vi "Rasnik_Gabri.vi"() -> ()   [LabVIEW 2015]
uses:
  GlobalPath.vi
  GlobalData.vi
  <vilib>/Utility/file.llb/Read Delimited Spreadsheet (string).vi
  <vilib>/Utility/file.llb/Write Delimited Spreadsheet (DBL).vi
panel:
  out "all rows 4":string[][](array[string])
  out "all rows 3":string[][](array[string])
  out "appended path 2":path
  in  "Done?":bool
  in  "Stage":string
  in  "driver off":bool caption="Disconnect the driver from the power supply"
  out "text":string
  out "PanelName":string
  out "appended path":path
  out "Y Diff10":dbl
  out "Y Diff9":dbl
  out "Y Diff8":dbl
  out "Y Diff7":dbl
  out "Y Diff6":dbl
  out "Y Diff5":dbl
  out "Y Diff4":dbl
  out "Y Diff3":dbl
  out "Y Diff2":dbl
  out "Y Diff1":dbl
  out "X Diff10":dbl
  out "X Diff9":dbl
  out "X Diff8":dbl
  out "X Diff7":dbl
  out "X Diff6":dbl
  out "X Diff5":dbl
  out "X Diff4":dbl
  out "X Diff3":dbl
  out "X Diff2":dbl
  out "X Diff1":dbl
  out "all rows":string[][](array[string])
  out "Y D10":dbl format="%.2f"
  out "Y D9":dbl format="%.2f"
  out "Y D8":dbl format="%.2f"
  out "Y D7":dbl format="%.2f"
  out "Y D6":dbl format="%.2f"
  out "Y D5":dbl format="%.2f"
  out "Y D4":dbl format="%.2f"
  out "Y D3":dbl format="%.2f"
  out "Y D2":dbl format="%.2f"
  out "Y D1":dbl
  out "X D10":dbl format="%.2f"
  out "X D9":dbl format="%.2f"
  out "X D8":dbl format="%.2f"
  out "X D7":dbl format="%.2f"
  out "X D6":dbl format="%.2f"
  out "X D5":dbl format="%.2f"
  out "X D4":dbl format="%.2f"
  out "X D3":dbl format="%.2f"
  out "X D2":dbl format="%.2f"
  out "X D1":dbl
  out "y 6":string
  out "y 10":string
  out "y 9":string
  out "y 8":string
  out "y 7":string
  out "y 5":string
  out "y 4":string
  out "y 3":string
  out "y 2":string
  out "y 1":string
  out "x 6":string
  out "x 10":string
  out "x 9":string
  out "x 8":string
  out "x 7":string
  out "x 5":string
  out "x 4":string
  out "x 3":string
  out "x 2":string
  out "x 1":string
  out "Script":path
  out "Filename selected":path
  out "standard output":string
  in  "Done?":bool
  in  "Open Program":bool
  in  "c-ccd 3":bool caption="Setup the electronics for the C-CCD reading:\n- make sure the ethernet cables are connected on the minimal heads\n- check that the cables connecting the driver with the muxs are plugged in\n- CONNECT the driver to the power supply and check that it is connected to the LAN\nIf the measurements show -1 in all c-ccds:\nUNPLUG the driver, WAIT a couple of seconds and REPLUG it"
  in  "c-ccd":bool caption="Read the data file"
  # "Rasmask reading from PCBs on stiffback/table"
  # "Type \"Table\" or \"Stiffback\" for the C-CCDs you want to use:"
  # "Run the C-CCD reading program \n(the 10 Rasmasks are automatically read and the data saved)"
  # "Data file reading"
  # "The most recent data file created by the C-CCD program will be opened.\nOnce the \"read data file\" is clicked, the raw data and displacement should appear on the PCB schematics on the bottom."
  # "Raw Data (mm):"
  # "Calibrated position (mm):"
  # "Difference (wrt Reference reading) (um):"
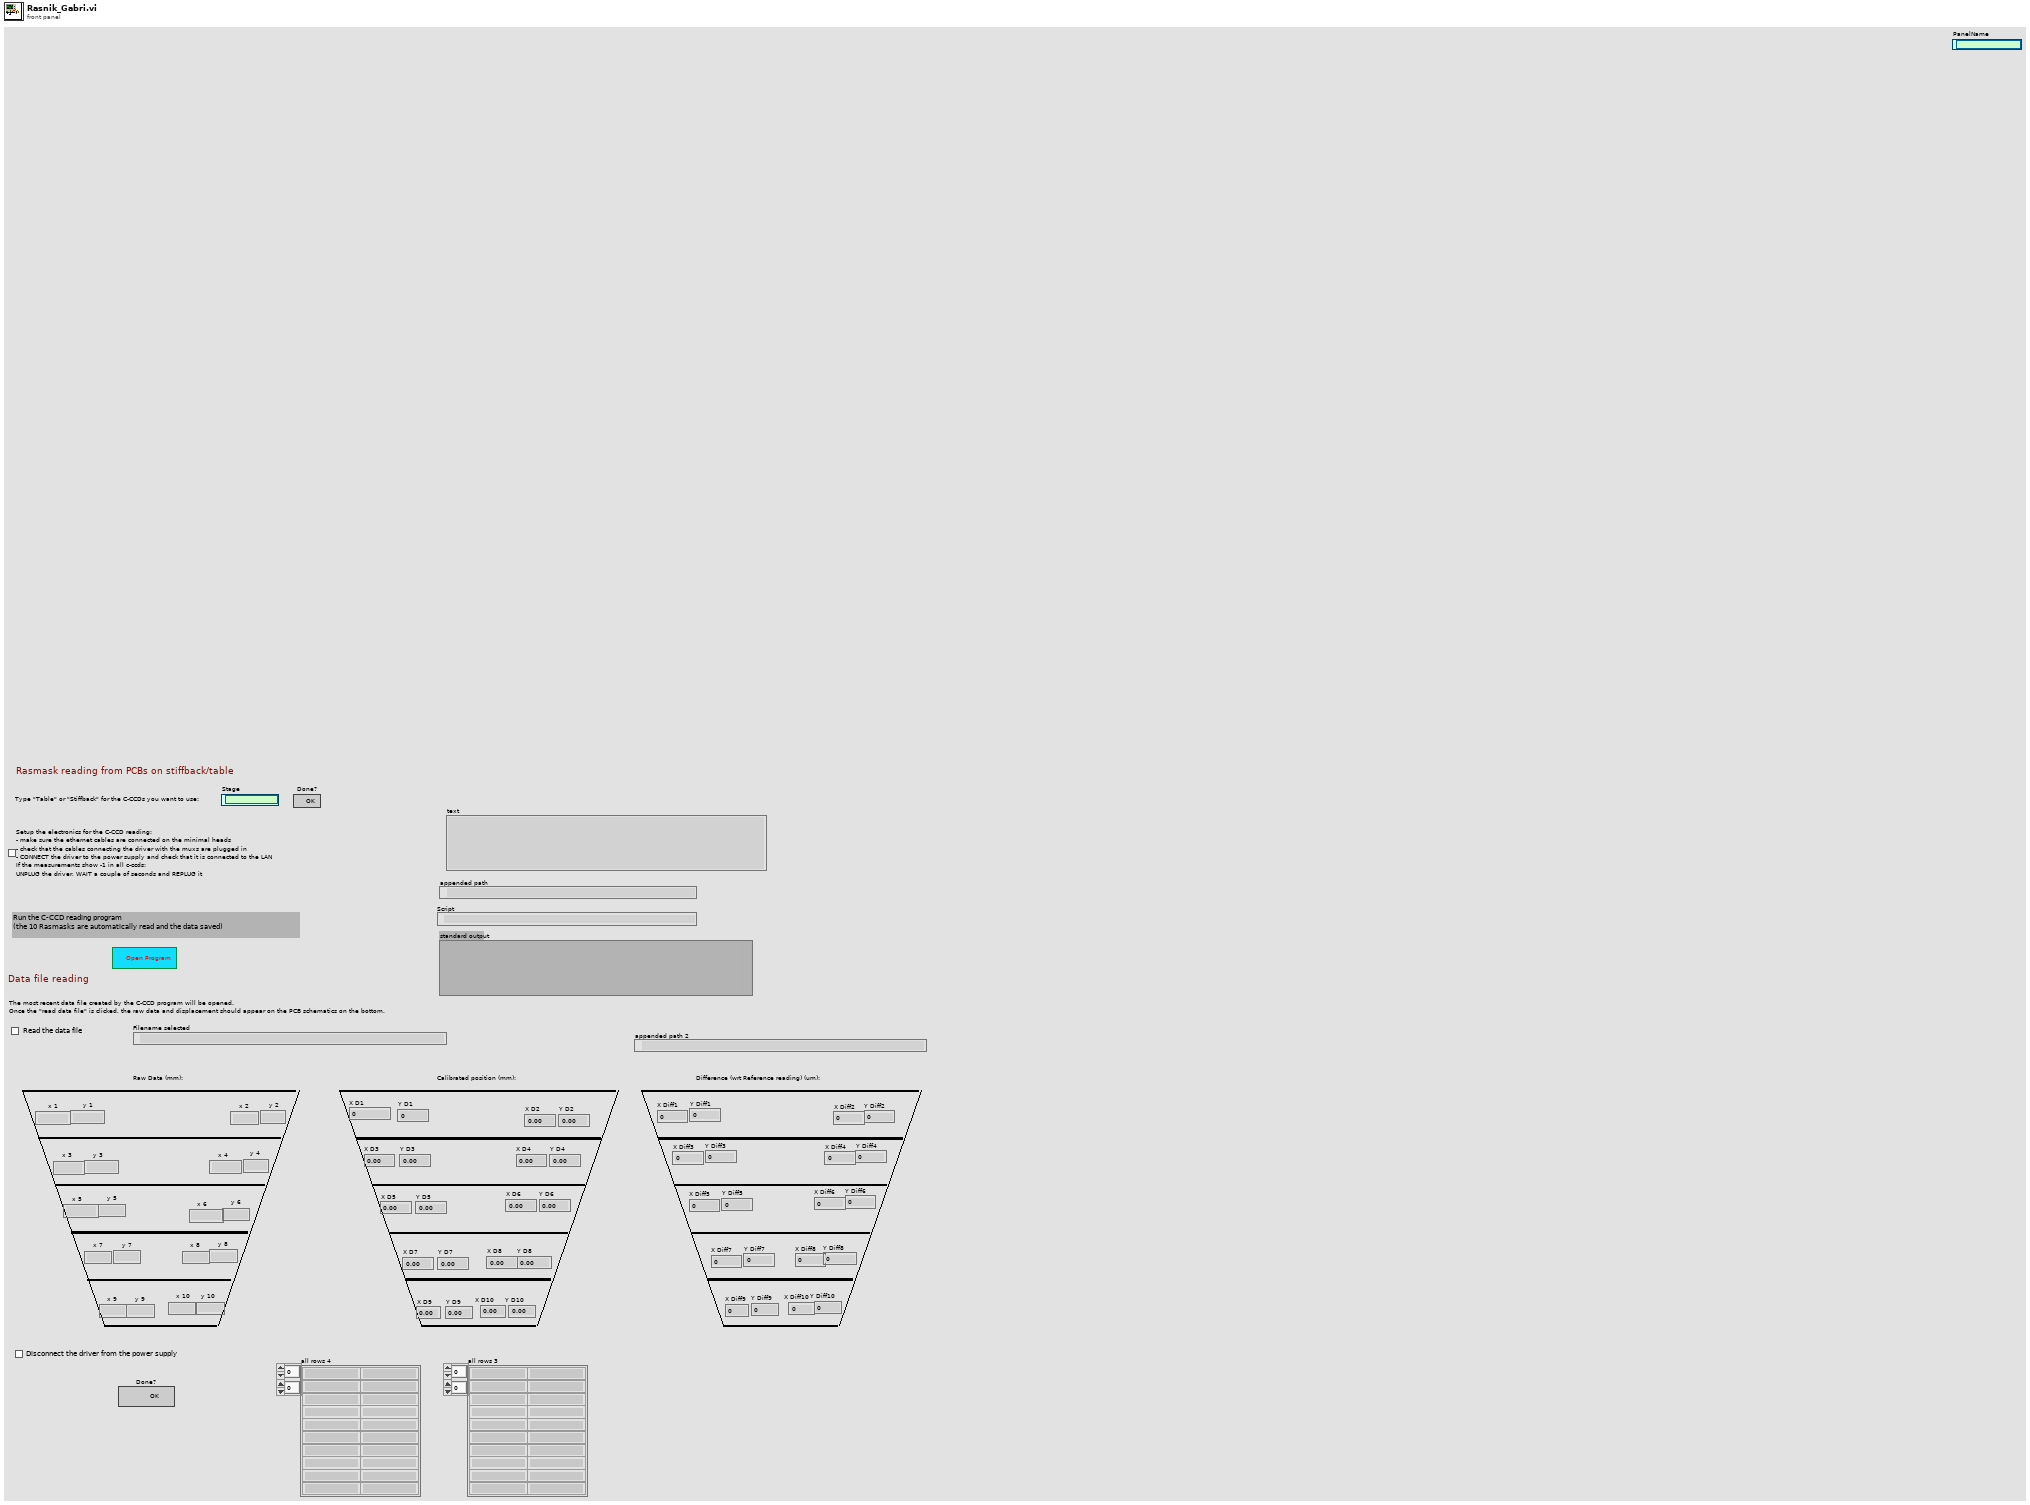
[diagram p1: front panel]
types:
  T1 = enum16{"open", "replace", "create", "open or create", "replace or create", "replace or create with confirmation"}
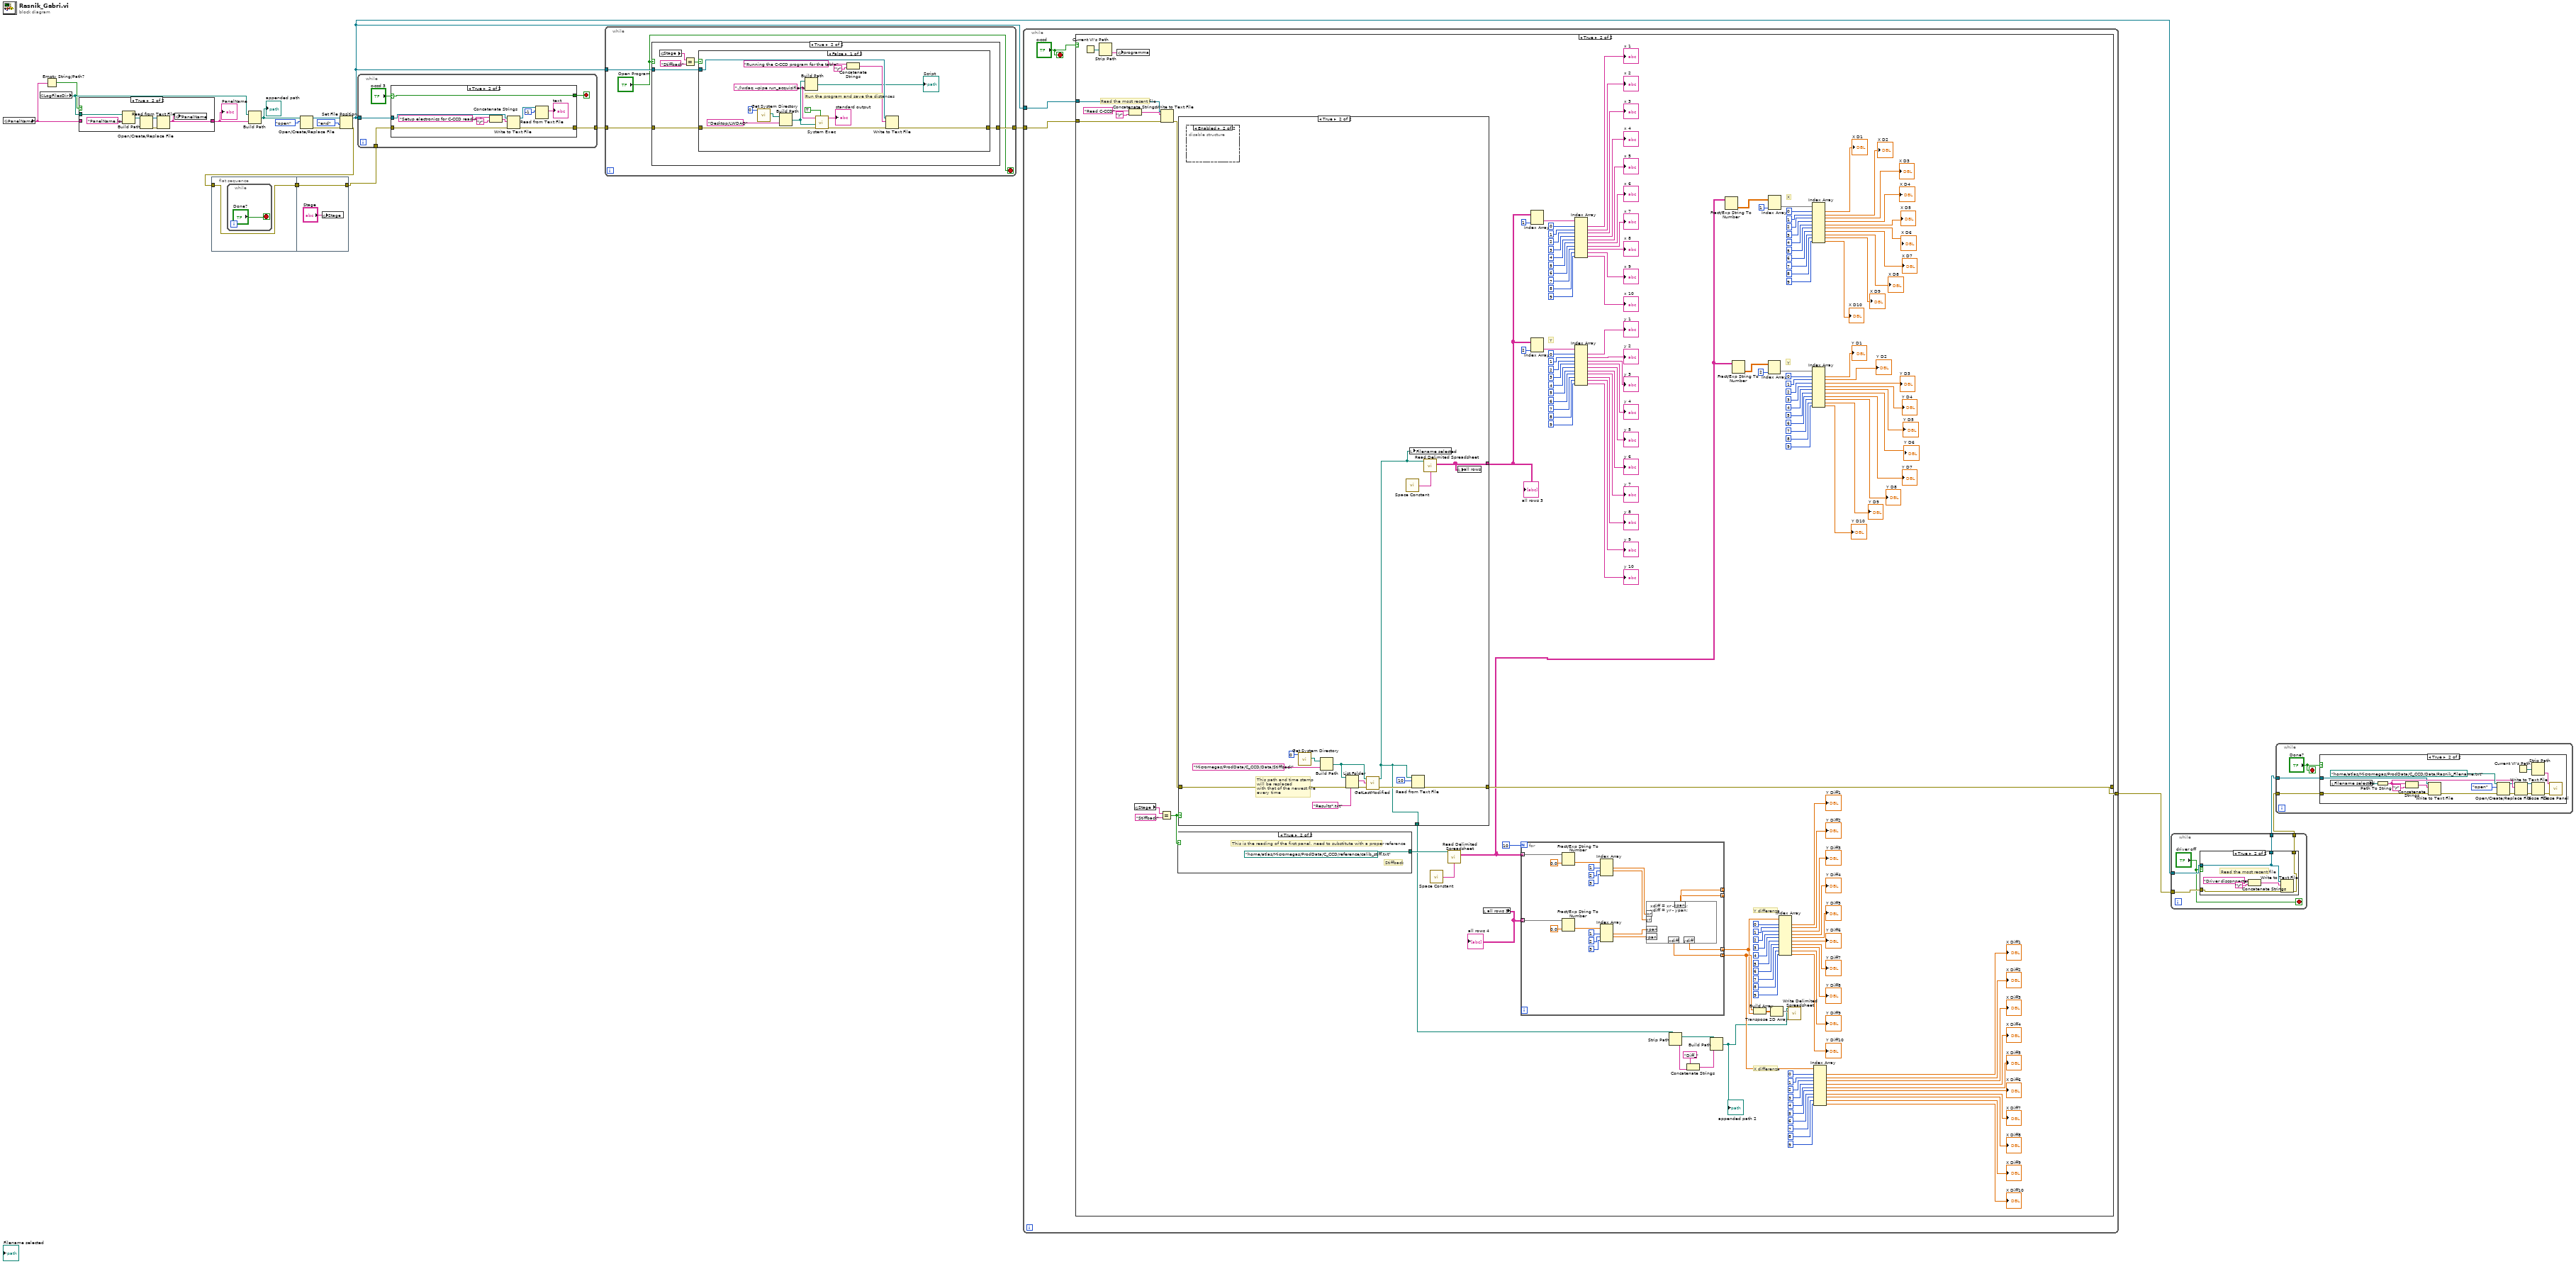
[diagram p0: block diagram]
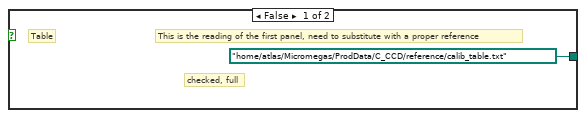
[diagram p5: hidden frame]
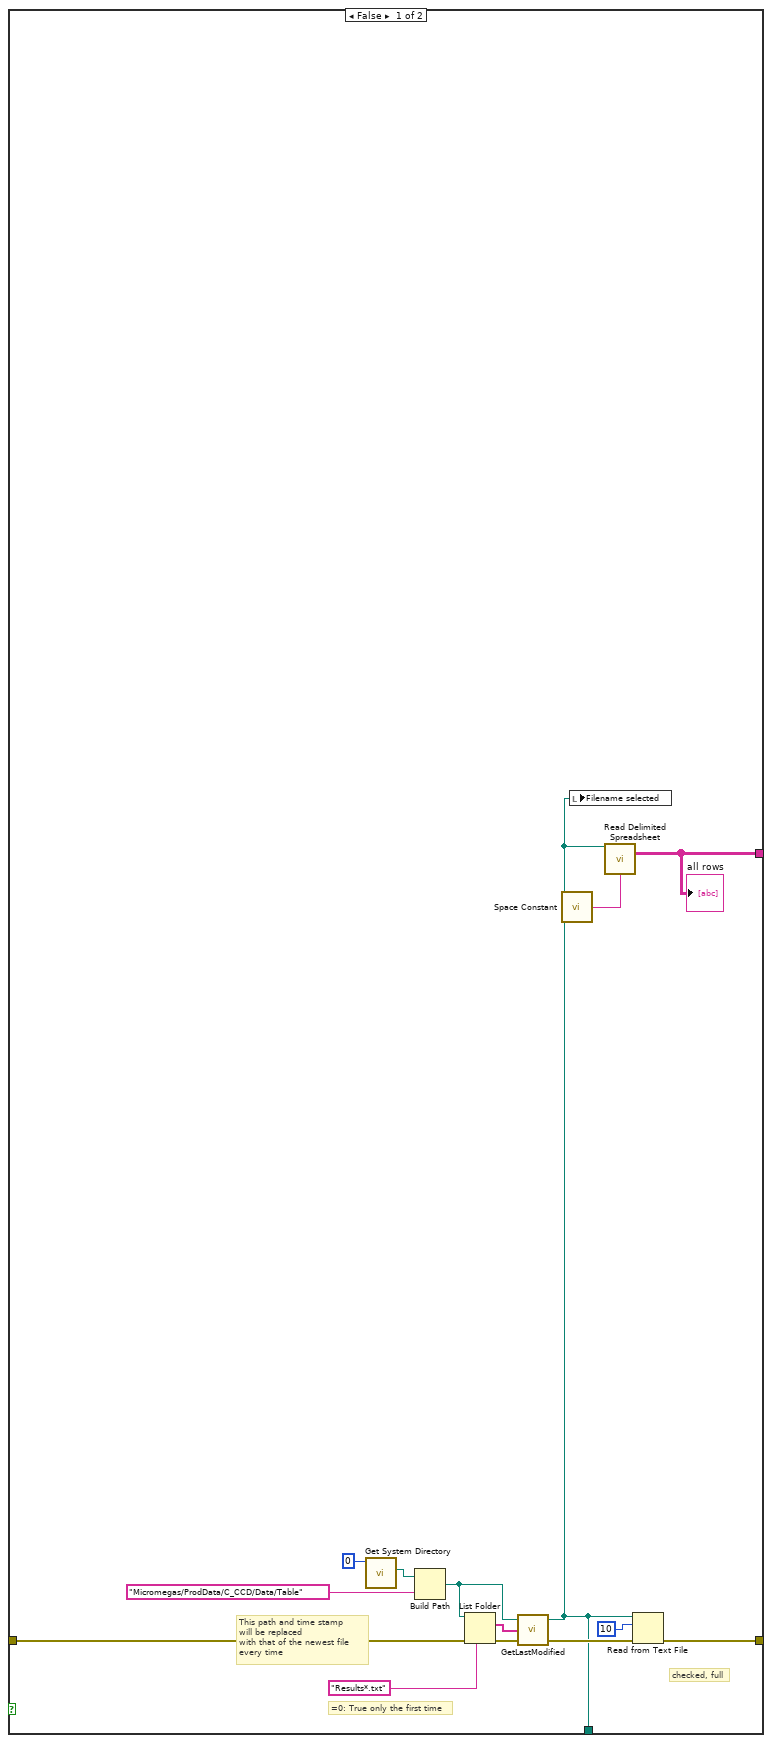
[diagram p6: hidden frame]
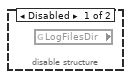
[diagram p7: hidden frame]
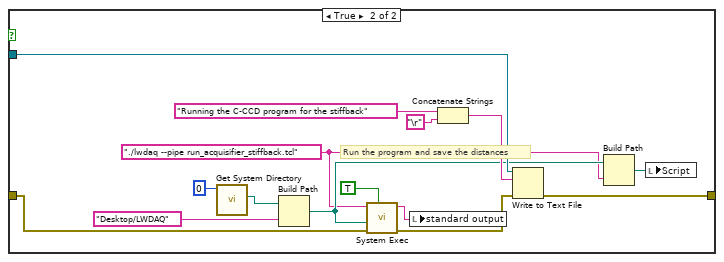
[diagram p10: hidden frame]
diagram:
  n1 = global read "GlobalData.vi" "PanelName"() -> (w14:string)
  n2 = global read "GlobalPath.vi" "LogFilesDir"() -> (w15:path)
  n3 = Empty String/Path?(string/path=w14) -> (empty?=w13:bool)
  n4 = case shown="True" w13 {
    tunnel: w15 -> [_ w25]
    tunnel: [w19 w20] -> w16
    tunnel: w14 -> [w19 _]
    frame False {
    }
    frame True {
      n5 = Build Path(base path=w25, name or relative path="PanelName.log") -> (appended path=w24:path)
      n6 = Open/Create/Replace File(file path (use dialog)=w24) -> (refnum out=w21:refnum<file>, error out=w22:errorcluster)  [unwired: 5 in, 1 out]
      n7 = Read from Text File(file (use dialog)=w21, error in=w22) -> (text=w20:string)  [unwired: 2 in, 3 out]
      n8 = global write "GlobalData.vi" "PanelName"(w20) -> ()
    }
  }
  "PanelName" <- w16
  n9 = flat-sequence {
    tunnel: w3 -> [w26]
    tunnel: [w26] -> w2
    tunnel: [w28] -> w1
    tunnel: w2 -> [w28]
    frame #0 {
      n10 = while {
        stop <- "Done?" stop-if-true
      }
    }
    frame #1 {
      n11 = global write "GlobalData.vi" "Stage"("Stage") -> ()
    }
  }
  n12 = Build Path(base path=w15, name or relative path=w16) -> (appended path=w8:path)
  "appended path" <- w8
  n13 = Open/Create/Replace File(file path (use dialog)=w8, operation (0:open)=T1."open") -> (refnum out=w11:refnum<file>, error out=w12:errorcluster)  [unwired: 4 in, 1 out]
  n14 = Set File Position(refnum=w11, from (0:start)=enum16{"start", "end", "current"}."end", error in=w12) -> (refnum out=w7:refnum<file>, error out=w3:errorcluster)  [unwired: 1 in]
  n15 = while {
    tunnel: w7 -> [w33]
    tunnel: [w31] -> w17
    tunnel: w1 -> [w30]
    stop <- w32 stop-if-true
    n16 = case shown="True" "c-ccd 3" {
      selector: "c-ccd 3" -> [w36 w43]
      tunnel: [w35 w44] -> w31
      tunnel: w33 -> [_ w41]
      tunnel: [w36 w43] -> w32
      tunnel: w30 -> [w35 w42]
      frame False {
      }
      frame True {
        n17 = Concatenate Strings("Setup electronics for C-CCD reading", "\r") -> (w40:string)
        n18 = Write to Text File(file (use dialog)=w41, text=w40, error in=w42) -> (refnum out=w39:refnum<file>, error out=w44:errorcluster)  [unwired: 1 in, 1 out]
        n19 = Read from Text File(file (use dialog)=w39, count=-1) -> (text=→"text":string)  [unwired: 2 in, 3 out]
      }
    }
  }
  n20 = while {
    tunnel: w7 -> [w48]
    tunnel: w17 -> [w50]
    tunnel: [w49] -> w18
    stop <- "Open Program" stop-if-true
    n21 = case shown="True" "Open Program" {
      tunnel: w50 -> [w51 w54]
      tunnel: [w51 w53] -> w49
      tunnel: w48 -> [_ w52]
      frame False {
      }
      frame True {
        n22 = global read "GlobalData.vi" "Stage"() -> (w56:string)
        n23 = Equal?(x=w56, y="Stiffback") -> (x = y?=w55:bool)
        n24 = case shown="False" w55 {
          tunnel: w54 -> [w69 w84]
          tunnel: [w67 w82] -> w53
          tunnel: w52 -> [w66 w81]
          frame False {
            w59 = "./lwdaq --pipe run_acquisifier.tcl"
            # "Run the program and save the distances"
            n25 = call <vilib>:"Get System Directory.vi"("system directory type"=0) -> ("system directory"=w64:path)  [unwired: 10 in]
            n26 = Build Path(base path=w64, name or relative path="Desktop/LWDAQ") -> (appended path=w60:path)
            n27 = Build Path(base path=w60, name or relative path=w59) -> (appended path=→"Script":path)
            n28 = call <vilib>:"System Exec.vi"("wait until completion? (T)"=TRUE, "error in (no error)"=w69, "working directory"=w60, "command line"=w59) -> ("error out"=w68:errorcluster, "standard output"=→"standard output":string)  [unwired: 4 in, 2 out]
            n29 = Concatenate Strings("Running the C-CCD program for the table", "\r") -> (w72:string)
            n30 = Write to Text File(file (use dialog)=w66, text=w72, error in=w68) -> (error out=w67:errorcluster)  [unwired: 1 in, 2 out]
          }
          frame True {
            w75 = "./lwdaq --pipe run_acquisifier_stiffback.tcl"
            # "Run the program and save the distances"
            n31 = call <vilib>:"Get System Directory.vi"("system directory type"=0) -> ("system directory"=w78:path)  [unwired: 10 in]
            n32 = Build Path(base path=w78, name or relative path="Desktop/LWDAQ") -> (appended path=w76:path)
            n33 = call <vilib>:"System Exec.vi"("wait until completion? (T)"=TRUE, "error in (no error)"=w84, "working directory"=w76, "command line"=w75) -> ("error out"=w83:errorcluster, "standard output"=w73:string)  [unwired: 4 in, 2 out]
            n34 = local write "standard output"(w73) -> ()
            n35 = Concatenate Strings("Running the C-CCD program for the stiffback", "\r") -> (w87:string)
            n36 = Write to Text File(file (use dialog)=w81, text=w87, error in=w83) -> (error out=w82:errorcluster)  [unwired: 1 in, 2 out]
            n37 = Build Path(base path=w76, name or relative path=w75) -> (appended path=w74:path)
            n38 = local write "Script"(w74) -> ()
          }
        }
      }
    }
  }
  n39 = while {
    tunnel: w7 -> [w89]
    tunnel: w18 -> [w91]
    tunnel: [w90] -> w6
    stop <- "c-ccd" stop-if-true
    n40 = case shown="True" "c-ccd" {
      tunnel: w91 -> [w92 w243]
      tunnel: [w92 w241] -> w90
      tunnel: w89 -> [_ w240]
      frame False {
      }
      frame True {
        # "X"
        # "Y"
        # "Y differenza"
        # "X differenza"
        # "Y"
        # "Read the most recent file"
        n41 = Current VI's Path() -> (path=w244:path)
        n42 = Strip Path(path=w244) -> (name=w245:string)  [unwired: 1 out]
        n43 = global write "GlobalData.vi" "programma"(w245) -> ()
        n44 = Concatenate Strings("Read C-CCD", "\r") -> (w250:string)
        n45 = global read "GlobalData.vi" "Stage"() -> (w246:string)
        n46 = Equal?(x=w246, y="Stiffback") -> (x = y?=w151:bool)
        n47 = Write to Text File(file (use dialog)=w240, text=w250, error in=w243) -> (error out=w242:errorcluster)  [unwired: 1 in, 2 out]
        n48 = case shown="True" w151 {
          tunnel: [path "/home/atlas/Micromegas/ProdData/C_CCD/reference/calib_table.txt" ("file path (dialog if empty)") path "/home/atlas/Micromegas/ProdData/C_CCD/reference/calib_stiff.txt" ("file path (dialog if empty)")] -> w195
          frame False {
            # "checked, full"
            # "This is the reading of the first panel, need to substitute with a proper reference"
            # "Table"
          }
          frame True {
            # "Stiffback"
            # "This is the reading of the first panel, need to substitute with a proper reference"
          }
        }
        n49 = case shown="True" w151 {
          tunnel: w242 -> [w276 w290]
          tunnel: [w285 w299] -> w241
          tunnel: [w274 w288] -> w216
          tunnel: [w273 w287] -> w94
          frame False {
            # "checked, full"
            # "=0: True only the first time"
            # "This path and time stamp\nwill be replaced\nwith that of the newest file \nevery time"
            n50 = call <vilib>:"Get System Directory.vi"("system directory type"=0) -> ("system directory"=w283:path)  [unwired: 10 in]
            n51 = Build Path(base path=w283, name or relative path="Micromegas/ProdData/C_CCD/Data/Table") -> (appended path=w278:path)
            n52 = List Folder(path=w278, pattern="Results*.txt", error in=w276) -> (filenames=w281:string[], error out=w279:errorcluster)  [unwired: 1 in, 2 out]
            n53 = call "GetLastModified.vi"("error in"=w279, "filenames"=w281, "SearchDir"=w278) -> ("error out"=w280:errorcluster, "Path"=w273:path)  [unwired: 1 out]
            n54 = call <vilib>:"Space Constant.vi"() -> ("String"=w275:string)
            n55 = local write "Filename selected"(w273) -> ()
            n56 = call-poly <vilib>:"Read Delimited Spreadsheet.vi"("file path (dialog if empty)"=w273, "delimiter (\\t)"=w275) -> ("all rows"=w274:string[][])  [unwired: 8 in, 5 out]
            "all rows" <- w274
            n57 = Read from Text File(file (use dialog)=w273, count=10, error in=w280) -> (error out=w285:errorcluster)  [unwired: 1 in, 3 out]
          }
          frame True {
            # "This path and time stamp\nwill be replaced\nwith that of the newest file \nevery time"
            n58 = disable-structure shown="Enabled" {
              frame Disabled {
                n59 = global read "GlobalPath.vi" "LogFilesDir"() -> ()  [unwired: 1 out]
              }
              frame Enabled {
              }
            }
            n60 = call <vilib>:"Get System Directory.vi"("system directory type"=0) -> ("system directory"=w297:path)  [unwired: 10 in]
            n61 = Build Path(base path=w297, name or relative path="Micromegas/ProdData/C_CCD/Data/Stiffback") -> (appended path=w293:path)
            n62 = List Folder(path=w293, pattern="Results*.txt", error in=w290) -> (filenames=w292:string[], error out=w291:errorcluster)  [unwired: 1 in, 2 out]
            n63 = call "GetLastModified.vi"("error in"=w291, "filenames"=w292, "SearchDir"=w293) -> ("error out"=w294:errorcluster, "Path"=w287:path)  [unwired: 1 out]
            n64 = call <vilib>:"Space Constant.vi"() -> ("String"=w289:string)
            n65 = local write "Filename selected"(w287) -> ()
            n66 = Read from Text File(file (use dialog)=w287, count=10, error in=w294) -> (error out=w299:errorcluster)  [unwired: 1 in, 3 out]
            n67 = call-poly <vilib>:"Read Delimited Spreadsheet.vi"("file path (dialog if empty)"=w287, "delimiter (\\t)"=w289) -> ("all rows"=w288:string[][])  [unwired: 8 in, 5 out]
            n68 = local write "all rows"(w288) -> ()
          }
        }
        "all rows 3" <- w216
        n69 = call <vilib>:"Space Constant.vi"() -> ("String"=w148:string)
        n70 = call-poly <vilib>:"Read Delimited Spreadsheet.vi"("file path (dialog if empty)"=w195, "delimiter (\\t)"=w148) -> ("all rows"=w112:string[][])  [unwired: 8 in, 5 out]
        n71 = local read "all rows 3"() -> (w93:string[][])
        "all rows 4" <- w93
        n72 = for {
          N: 10 -> [_]
          tunnel: w112 -> [w270] mode=indexing
          tunnel: w93 -> [w269] mode=indexing
          tunnel: [w258] -> w173 mode=indexing
          tunnel: [w257] -> w152 mode=indexing
          tunnel: [w254] -> _ mode=indexing
          tunnel: [w253] -> _ mode=indexing
          n73 = Fract/Exp String To Number(string=w270, default (0 dbl)=0.0 ("default (0 DBL)")) -> (number=w272:dbl[])  [unwired: 2 in, 1 out]
          n74 = Fract/Exp String To Number(string=w269, default (0 dbl)=0.0 ("default (0 DBL)")) -> (number=w271:dbl[])  [unwired: 2 in, 1 out]
          n75 = Index Array(array=w272, index #1=1, index #2=2, index #3=3) -> (element #1=w262:dbl, element #2=w261:dbl)  [unwired: 1 out]
          n76 = Index Array(array=w271, index #1=1, index #2=2, index #3=3) -> (element #1=w259:dbl, element #2=w260:dbl)  [unwired: 1 out]
          n77 = formula code="xdiff = xr - xpan;\nydiff = yr - ypan;"("xr"=w262, "yr"=w261, "xpan"=w259, "ypan"=w260) -> ("xdiff"=w258:dbl, "ydiff"=w257:dbl, "xr"=w254:dbl, "xpan"=w253:dbl)
        }
        n78 = Index Array(array=w216, index (col)=1 ("disabled index (col)")) -> (element=w238:string[])  [unwired: 1 in]
        n79 = Index Array(array=w216, index (col)=2 ("disabled index (col)")) -> (element=w205:string[])  [unwired: 1 in]
        n80 = Index Array(array=w238, index #1=0, index #2=1, index #3=2, index #4=3, index #5=4, index #6=5, index #7=6, index #8=7, index #9=8, index #10=9) -> (element #1=→"x 1":string, element #2=→"x 2":string, element #3=→"x 3":string, element #4=→"x 4":string, element #5=→"x 5":string, element #6=→"x 6":string, element #7=→"x 7":string, element #8=→"x 8":string, element #9=→"x 9":string, element #10=→"x 10":string)
        n81 = Index Array(array=w205, index #1=0, index #2=1, index #3=2, index #4=3, index #5=4, index #6=5, index #7=6, index #8=7, index #9=8, index #10=9) -> (element #1=→"y 1":string, element #2=→"y 2":string, element #3=→"y 3":string, element #4=→"y 4":string, element #5=→"y 5":string, element #6=→"y 6":string, element #7=→"y 7":string, element #8=→"y 8":string, element #9=→"y 9":string, element #10=→"y 10":string)
        n82 = Strip Path(path=w94) -> (stripped path=w99:path, name=w98:string)
        n83 = Concatenate Strings("Diff_" ("string"), w98) -> (w96:string)
        n84 = Build Path(base path=w99, name or relative path=w96) -> (appended path=w95:path)
        "appended path 2" <- w95
        n85 = Fract/Exp String To Number(string=w112) -> (number=w124:dbl[][])  [unwired: 3 in, 1 out]
        n86 = Fract/Exp String To Number(string=w112) -> (number=w111:dbl[][])  [unwired: 3 in, 1 out]
        n87 = Build Array(w173, w152) -> (w149:dbl[][])
        n88 = Index Array(array=w111, index (col)=2 ("disabled index (col)")) -> (element=w110:dbl[])  [unwired: 1 in]
        n89 = Index Array(array=w124, index (col)=1 ("disabled index (col)")) -> (element=w123:dbl[])  [unwired: 1 in]
        n90 = Transpose 2D Array(2D array=w149) -> (transposed array=w147:dbl[][])
        n91 = Index Array(array=w152, index #1=0, index #2=1, index #3=2, index #4=3, index #5=4, index #6=5, index #7=6, index #8=7, index #9=8, index #10=9) -> (element #1=→"Y Diff1":dbl, element #2=→"Y Diff2":dbl, element #3=→"Y Diff3":dbl, element #4=→"Y Diff4":dbl, element #5=→"Y Diff5":dbl, element #6=→"Y Diff6":dbl, element #7=→"Y Diff7":dbl, element #8=→"Y Diff8":dbl, element #9=→"Y Diff9":dbl, element #10=→"Y Diff10":dbl)
        n92 = call-poly <vilib>:"Write Delimited Spreadsheet.vi"("file path (dialog if empty)"=w95, "2D data"=w147) -> ()  [unwired: 12 in, 2 out]
        n93 = Index Array(array=w110, index #1=0, index #2=1, index #3=2, index #4=3, index #5=4, index #6=5, index #7=6, index #8=7, index #9=8, index #10=9) -> (element #1=→"Y D1":dbl, element #2=→"Y D2":dbl, element #3=→"Y D3":dbl, element #4=→"Y D4":dbl, element #5=→"Y D5":dbl, element #6=→"Y D6":dbl, element #7=→"Y D7":dbl, element #8=→"Y D8":dbl, element #9=→"Y D9":dbl, element #10=→"Y D10":dbl)
        n94 = Index Array(array=w123, index #1=0, index #2=1, index #3=2, index #4=3, index #5=4, index #6=5, index #7=6, index #8=7, index #9=8, index #10=9) -> (element #1=→"X D1":dbl, element #2=→"X D2":dbl, element #3=→"X D3":dbl, element #4=→"X D4":dbl, element #5=→"X D5":dbl, element #6=→"X D6":dbl, element #7=→"X D7":dbl, element #8=→"X D8":dbl, element #9=→"X D9":dbl, element #10=→"X D10":dbl)
        n95 = Index Array(array=w173, index #1=0, index #2=1, index #3=2, index #4=3, index #5=4, index #6=5, index #7=6, index #8=7, index #9=8, index #10=9) -> (element #1=→"X Diff1":dbl, element #2=→"X Diff2":dbl, element #3=→"X Diff3":dbl, element #4=→"X Diff4":dbl, element #5=→"X Diff5":dbl, element #6=→"X Diff6":dbl, element #7=→"X Diff7":dbl, element #8=→"X Diff8":dbl, element #9=→"X Diff9":dbl, element #10=→"X Diff10":dbl)
      }
    }
  }
  n96 = while {
    tunnel: w7 -> [w305]
    tunnel: w6 -> [w304]
    tunnel: [w303] -> w5
    tunnel: [w302] -> w4
    stop <- "driver off" stop-if-true
    n97 = case shown="True" "driver off" {
      tunnel: w305 -> [w307 w309]
      tunnel: w304 -> [w306 w310]
      tunnel: [w307 w309] -> w303
      tunnel: [w306 w308] -> w302
      frame False {
      }
      frame True {
        # "Read the most recent file"
        n98 = Concatenate Strings("Driver disconnected", "\r") -> (w313:string)
        n99 = Write to Text File(file (use dialog)=w309, text=w313, error in=w310) -> (error out=w308:errorcluster)  [unwired: 1 in, 2 out]
      }
    }
  }
  n100 = while {
    tunnel: w4 -> [w315]
    tunnel: w5 -> [w314]
    stop <- "Done?" stop-if-true
    n101 = case shown="True" "Done?" {
      tunnel: w315 -> [_ w320]
      tunnel: w314 -> [_ w319]
      frame False {
      }
      frame True {
        n102 = local read "Filename selected"() -> (w321:path)
        n103 = Path To String(path=w321) -> (string=w327:string)
        n104 = Concatenate Strings(w327, "\r") -> (w328:string)
        n105 = Write to Text File(file (use dialog)=w319, text=w328, error in=w320) -> (error out=w317:errorcluster)  [unwired: 1 in, 2 out]
        n106 = Open/Create/Replace File(file path (use dialog)=path "/home/atlas/Micromegas/ProdData/C_CCD/Data/Rasnik_Filename.txt", error in=w317, operation (0:open)=T1."open") -> (refnum out=w326:refnum<file>, error out=w323:errorcluster)  [unwired: 3 in, 1 out]
        n107 = Write to Text File(file (use dialog)=w326, text=w327, error in=w323) -> (refnum out=w325:refnum<file>, error out=w324:errorcluster)  [unwired: 1 in, 1 out]
        n108 = Current VI's Path() -> (path=w331:path)
        n109 = Strip Path(path=w331) -> (name=w332:string)  [unwired: 1 out]
        n110 = Close File(refnum=w325, error in=w324) -> (error out=w318:errorcluster)  [unwired: 1 out]
        n111 = call <vilib>:"Close Panel.vi"("error in (no error)"=w318, "VI name"=w332) -> ()  [unwired: 9 in, 1 out]
      }
    }
  }
